vi "Close Actor Core Ref.vi"(8 "error in (no error)":errorcluster, 11 "Actor in":refnum<class "Actor.lvclass">) -> (0 "error out":errorcluster, 3 "Actor out":refnum<class "Actor.lvclass">)   [LabVIEW 2017, in "IViewable.lvlib" / "IViewable.lvclass"]
doc: "<License>\nCopyright © 2017 Composed Systems, LLC | All rights reserved\nwww.composed.io\n\nAuthor: Ethan Stern <ethan.stern@composed.io>\n\nThis software is provided \"AS IS\" WITHOUT WARRANTIES, either express or implied, AND IS FOR EDUCATIONAL PURPOSES ONLY.\n</License>"
uses:
  <vilib>/gpm_packages/@cs/mva-viewable/Source/IViewable/IViewable/IViewable.lvclass
  <vilib>/ActorFramework/Actor/Actor.lvclass
  C:/Program Files/National Instruments/LabVIEW 2017/vi.lib/ActorFramework/Actor/Actor.lvclass
  <vilib>/gpm_packages/@cs/mva-viewable/Source/IViewable/IViewable/IViewable.lvclass/IViewable.ctl
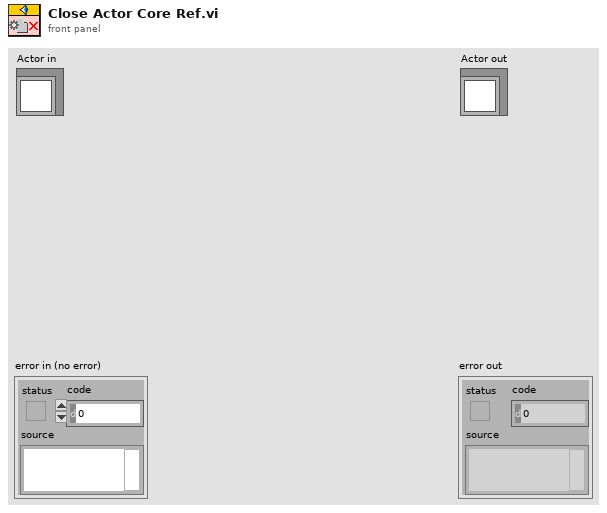
[diagram p1: front panel]
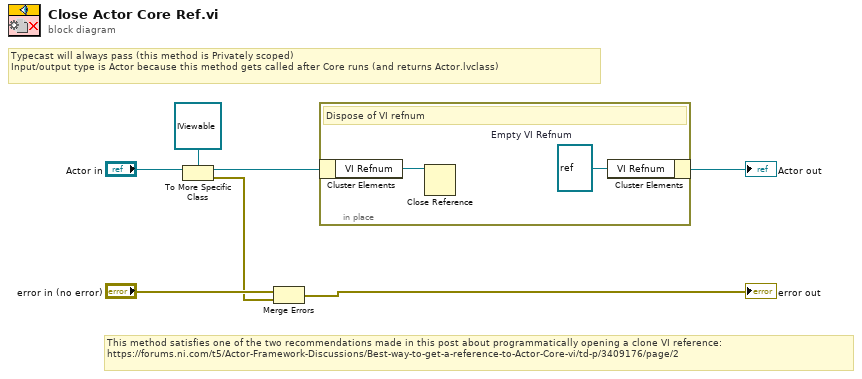
[diagram p0: block diagram]
diagram:
  # "Typecast will always pass (this method is Privately scoped)\nInput/output type is Actor because this method gets called after Core runs (and returns Actor.lvclass)"
  # "This method satisfies one of the two recommendations made in this post about programmatically opening a clone VI reference:\nhttps://forums.ni.com/t5/Actor-Framework-Discussions/Best-way-to-get-a-reference-to-Actor-Core-vi/td-p/3409176/page/2"
  n1 = To More Specific Class(target class=refnum<class "IViewable.lvclass"> refnum ("IViewable.lvlib:IViewable.lvclass"), reference="Actor in") -> (specific class reference=w2:refnum<class "IViewable.lvclass">, error out=w3:errorcluster)  [unwired: 1 in]
  n2 = Merge Errors("error in (no error)", w3) -> (→"error out":errorcluster)
  n3 = in-place {
    w8 = refnum<vi> refnum  # Empty VI Refnum
    # "Dispose of VI refnum"
    n4 = in-place-cluster #1(w2) -> ("VI Refnum"=w9:refnum<vi>)
    n5 = Close Reference(reference=w9) -> ()  [unwired: 1 in, 1 out]
    n6 = in-place-cluster #1("VI Refnum"=w8) -> (→"Actor out":refnum<class "IViewable.lvclass">)
  }
